vi "GetVisionTarget.vi"() -> (13 "Vision Timestamp (ms)":u32, 14 "Vision Horizontal Angle to Target (deg) [t-?]":dbl, 15 "Vision Vertical Angle to Target (deg) [t-?]":dbl, 16 "Vision Target Valid [t-?]":bool)   [LabVIEW 2020]
doc: "Reads the raw data from the LimeLight used for targeting the HUB. Performs some minor transformations and conducts intial validity checks."
uses:
  2d64956e-cf35-4d84-838e-e30eff74bf58.vi
  <vilib>/Rock Robotics/Network Tables/NT Read Number.vi
  GlobalDriverStationData.vi
  sensordata.vi
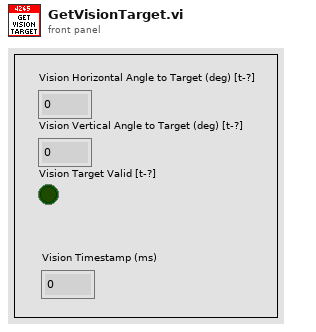
[diagram p1: front panel]
types:
  T1 = enum16{"Boot Up", "Camera Override", "HUB Targeting", "CARGO Tracking"}
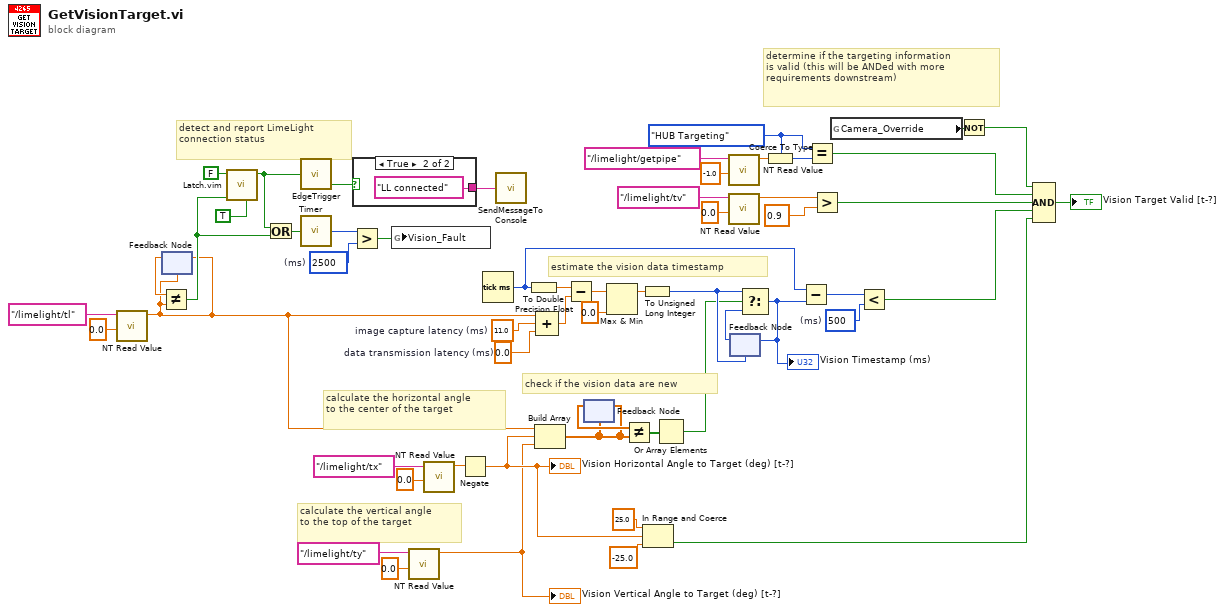
[diagram p0: block diagram]
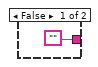
[diagram p2: hidden frame]
diagram:
  w7 = 0.0  # data transmission latency (ms)
  w18 = u32 2500  # (ms)
  w2 = u32 500  # (ms)
  w37 = 11.0  # image capture latency (ms)
  w42 = T1."HUB Targeting" ("x")
  # "detect and report LimeLight\nconnection status"
  # "calculate the horizontal angle\nto the center of the target"
  # "determine if the targeting information\nis valid (this will be ANDed with more\nrequirements downstream)"
  # "calculate the vertical angle\nto the top of the target"
  # "estimate the vision data timestamp"
  # "check if the vision data are new"
  n1 = call-poly <vilib>:"NT Read Value.vi"("Default Value"=0.0, "Name"="/limelight/tl") -> ("Numeric"=w4:dbl)  [unwired: 8 in, 1 out]
  n2 = feedback-in #1(w4) -> ()
  n3 = feedback #1(w4) -> (w20:dbl)
  n4 = Not Equal?(x=w20, y=w4) -> (x != y?=w15:bool)
  n5 = call "Latch.vim"("Default Value"=TRUE, "Latch Signal"=w15, "Latch Value"=FALSE) -> ("Latched"=w13:bool)  [unwired: 8 in]
  n6 = Or(x=w13, y=w15) -> (x .or. y?=w17:bool)
  n7 = call "EdgeTrigger.vi"("Input Signal"=w13) -> ("Falling Edge Trigger"=w11:bool)  [unwired: 2 out]
  n8 = call "Timer.vi"("Reset Timer"=w17) -> ("Time (ms)"=w19:u32)
  n9 = Greater?(x=w19, y=w18) -> (0:w1:bool)
  n10 = case shown="True" w11 {
    tunnel: ["" "LL connected" ("Message")] -> w12
    frame False {
    }
    frame True {
    }
  }
  n11 = global write "sensordata.vi" "Vision_Fault"(w1) -> ()
  n12 = call-poly <vilib>:"NT Read Value.vi"("Default Value"=0.0, "Name"="/limelight/ty") -> ("Numeric"=w3:dbl)  [unwired: 8 in, 1 out]
  "Vision Vertical Angle to Target (deg) [t-?]" <- w3
  n13 = call-poly <vilib>:"NT Read Value.vi"("Default Value"=0.0, "Name"="/limelight/tx") -> ("Numeric"=w48:dbl)  [unwired: 8 in, 1 out]
  n14 = Negate(x=w48) -> (-x=w5:dbl)
  "Vision Horizontal Angle to Target (deg) [t-?]" <- w5
  n15 = Tick Count (ms)() -> (millisecond timer value=w25:u32)
  n16 = call "SendMessageToConsole.vi"("Message String"=w12) -> ()  [unwired: 1 in]
  n17 = To Double Precision Float(number=w25) -> (double precision float=w35:dbl)
  n18 = Build Array(w4, w5, w3) -> (w29:dbl[])
  n19 = Compound Arithmetic op=ADD(w4, w37, w7) -> (w36:dbl)
  n20 = Subtract(x=w35, y=w36) -> (x-y=w34:dbl)
  n21 = feedback-in #2(w29) -> ()
  n22 = feedback #2(w29) -> (w30:dbl[])
  n23 = Max & Min(x=w34, y=0.0) -> (max(x,y)=w32:dbl)  [unwired: 1 out]
  n24 = Not Equal?(x=w30, y=w29) -> (x != y?=w28:bool[])
  n25 = To Unsigned Long Integer(number=w32) -> (unsigned 32bit integer=w31:u32)
  n26 = In Range and Coerce(upper limit=25.0, x=w5, lower limit=-25.0) -> (In Range?=w8:bool)  [unwired: 1 out]
  n27 = Or Array Elements(Boolean array=w28) -> (logical OR=w27:bool)
  n28 = call-poly <vilib>:"NT Read Value.vi"("Default Value"=-1.0, "Name"="/limelight/getpipe") -> ("Numeric"=w45:dbl)  [unwired: 8 in, 1 out]
  n29 = call-poly <vilib>:"NT Read Value.vi"("Default Value"=0.0, "Name"="/limelight/tv") -> ("Numeric"=w52:dbl)  [unwired: 8 in, 1 out]
  n30 = feedback #3(w31) -> (w38:u32)
  n31 = Select(t=w31, s=w27, f=w38) -> (s? t:f=w26:u32)
  "Vision Timestamp (ms)" <- w26
  n32 = feedback-in #3(w26) -> ()
  n33 = Coerce To Type(0:w45, 1:w42) -> (2:w44:T1)
  n34 = Subtract(x=w25, y=w26) -> (x-y=w24:u32)
  n35 = Equal?(x=w42, y=w44) -> (x = y?=w43:bool)
  n36 = Greater?(x=w52, y=0.9) -> (0:w41:bool)
  n37 = global read "GlobalDriverStationData.vi" "Camera_Override"() -> (w22:bool)
  n38 = Less?(x=w24, y=w2) -> (x < y?=w23:bool)
  n39 = Not(x=w22) -> (.not. x?=w21:bool)
  n40 = Compound Arithmetic op=AND(w21, w43, w41, w23, w8) -> (→"Vision Target Valid [t-?]":bool)
